vi "split_wavechannels (SubVI).vi"(8 "Sample rate":dbl, 11 "Array in":dbl[](array[numeric])) -> (3 "Array out":waveform(dbl)[](array[waveform]))   [LabVIEW 2021]
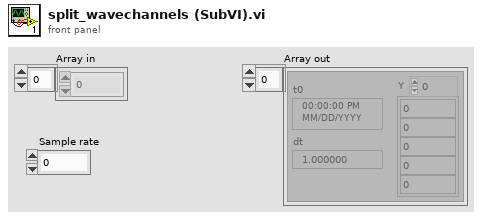
[diagram p1: front panel]
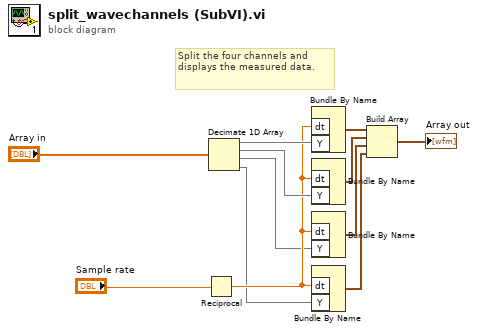
[diagram p0: block diagram]
diagram:
  # "Split the four channels and displays the measured data."
  n1 = Reciprocal(x="Sample rate") -> (1/x=w6:dbl)
  n2 = Decimate 1D Array("Array in") -> (w8:dbl[], w7:dbl[], w5:dbl[], w2:dbl[])
  n3 = Bundle By Name("dt"=w6, "Y"=w8) -> (w10:waveform(dbl))  [unwired: 1 out]
  n4 = Bundle By Name("dt"=w6, "Y"=w7) -> (w11:waveform(dbl))  [unwired: 1 out]
  n5 = Bundle By Name("dt"=w6, "Y"=w5) -> (w4:waveform(dbl))  [unwired: 1 out]
  n6 = Bundle By Name("dt"=w6, "Y"=w2) -> (w3:waveform(dbl))  [unwired: 1 out]
  n7 = Build Array(w10, w11, w4, w3) -> (→"Array out":waveform(dbl)[])
